vi "Construct.vi"(8 "error in":errorcluster, 10 "hardware configuration file on target":path, 11 "device parameters":T1) -> (0 "error out":errorcluster, 3 "Ballard ARINC-429 shared resources out":refnum<class "Ballard ARINC-429 Shared Resources.lvclass">)   [LabVIEW 2020, in "Ballard ARINC 429 Engine.lvlib" / "Implementation.lvlib" / "Ballard ARINC-429 Shared Resources.lvclass"]
uses:
  Ballard ARINC-429 Shared Resources.lvclass
  Shared/Device Parameters.ctl
  Shared/Initialization Method.ctl
  Ballard ARINC-429 Shared Resources.lvclass/Ballard ARINC-429 Shared Resources.ctl
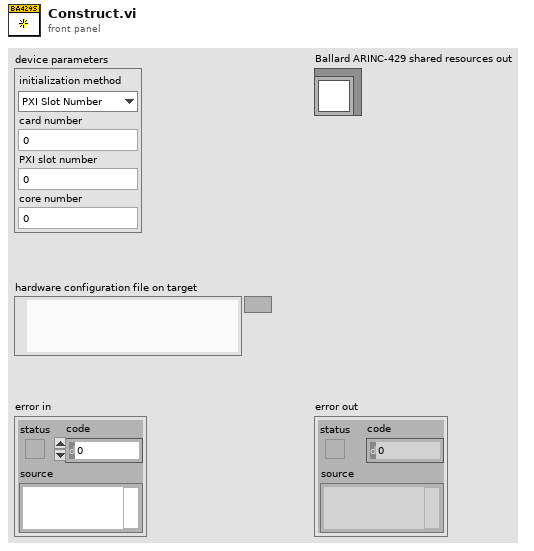
[diagram p1: front panel]
types:
  T1 = typedef "Device Parameters.ctl" = cluster{"initialization method":T2, "card number":i32, "PXI slot number":i32, "core number":i32}
  T2 = typedef "Initialization Method.ctl" = enum16{"PXI Slot Number", "Card Number"}
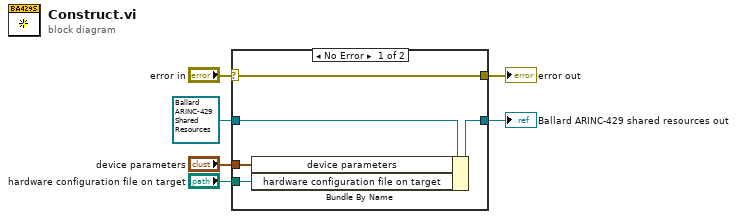
[diagram p0: block diagram]
diagram:
  n1 = case shown="No Error" "error in" {
    selector: "error in" -> [w11 w13]
    tunnel: [w11 w13] -> w5
    tunnel: [w7 w12] -> w4
    tunnel: refnum<class "Ballard ARINC-429 Shared Resources.lvclass"> refnum ("Ballard ARINC-429 Shared Resources out") -> [w10 w12]
    tunnel: "device parameters" -> [w9 _]
    tunnel: "hardware configuration file on target" -> [w8 _]
    frame No Error {
      n2 = Bundle By Name(cluster=w10, "device parameters"=w9, "hardware configuration file on target"=w8) -> (w7:refnum<class "Ballard ARINC-429 Shared Resources.lvclass">)
    }
    frame Error {
    }
  }
  "error out" <- w5
  "Ballard ARINC-429 shared resources out" <- w4
